vi "GetChanCrntSts.vi"(8 "错误输入（无错误）":errorcluster, 11 "设备中活动通道":u8) -> (0 "错误输出":errorcluster, 3 "返回值":i32)   [LabVIEW 2014]
uses:
  X86Dll/ZXUTConfigMgr.dll
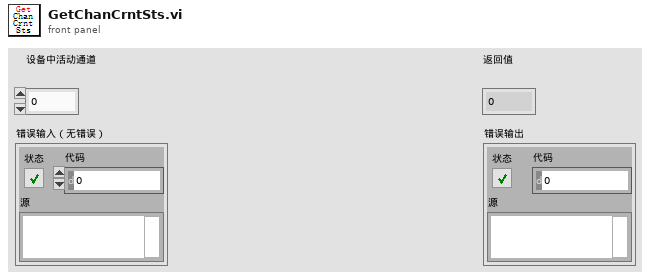
[diagram p1: front panel]
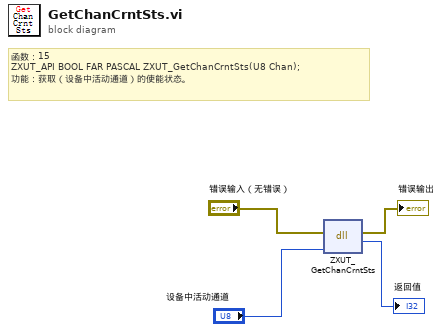
[diagram p0: block diagram]
diagram:
  # "函数：15\nZXUT_API BOOL\tFAR PASCAL ZXUT_GetChanCrntSts(U8 Chan);\n功能：获取（设备中活动通道）的使能状态。"
  n1 = dll-call lib="D:/Software/Utrasonic on-line monitoring/X86Dll/ZXUTConfigMgr.dll" fn="ZXUT_GetChanCrntSts"(error in="错误输入（无错误）", "Chan"="设备中活动通道") -> (error out=→"错误输出":errorcluster, "返回类型"=→"返回值":i32)  [unwired: 3 in, 1 out]
